vi "ThisLevelClassName.vi"(11 "SMO":refnum<class "SMO.lvclass">) -> (2 "Level class name":string, 3 "SMO out":refnum<class "SMO.lvclass">)   [LabVIEW 2019, in "SMO.lvclass"]
doc: "JKI State Machine Objects (SMO) 1.3.0.56\nJKI - JKI\nCopyright (c) 2017, JKI"
uses:
  SMO.lvclass
  <vilib>/regexp/Match Regular Expression.xnode
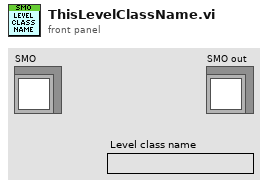
[diagram p1: front panel]
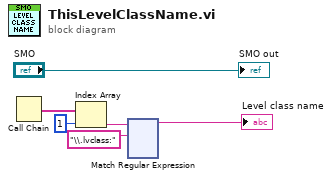
[diagram p0: block diagram]
diagram:
  n1 = Call Chain() -> (call chain=w6:string[])
  n2 = Index Array(array=w6, index=1) -> (element=w5:string)
  n3 = xnode "Match Regular Expression"("input string"=w5, "regular expression"="\\.lvclass:") -> ("before match"=→"Level class name":string)  [unwired: 4 in, 4 out]
  "SMO out" <- "SMO"
